vi "Solution part 1.vi"(11 "data?":bool) -> (3 "Occupied seats (result)":i16)   [LabVIEW 2020]
panel:
  out "Rounds":i32
  out "Seats":string[](array[string])
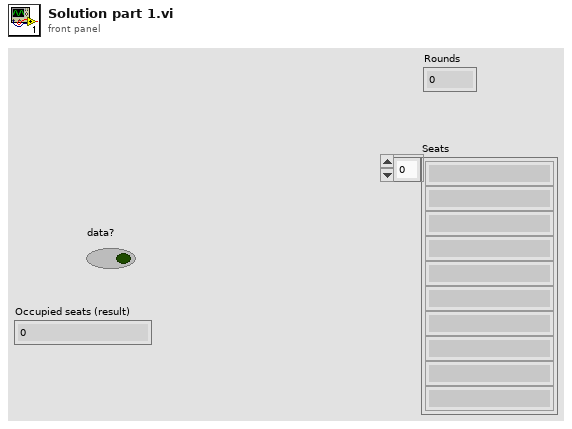
[diagram p1: front panel]
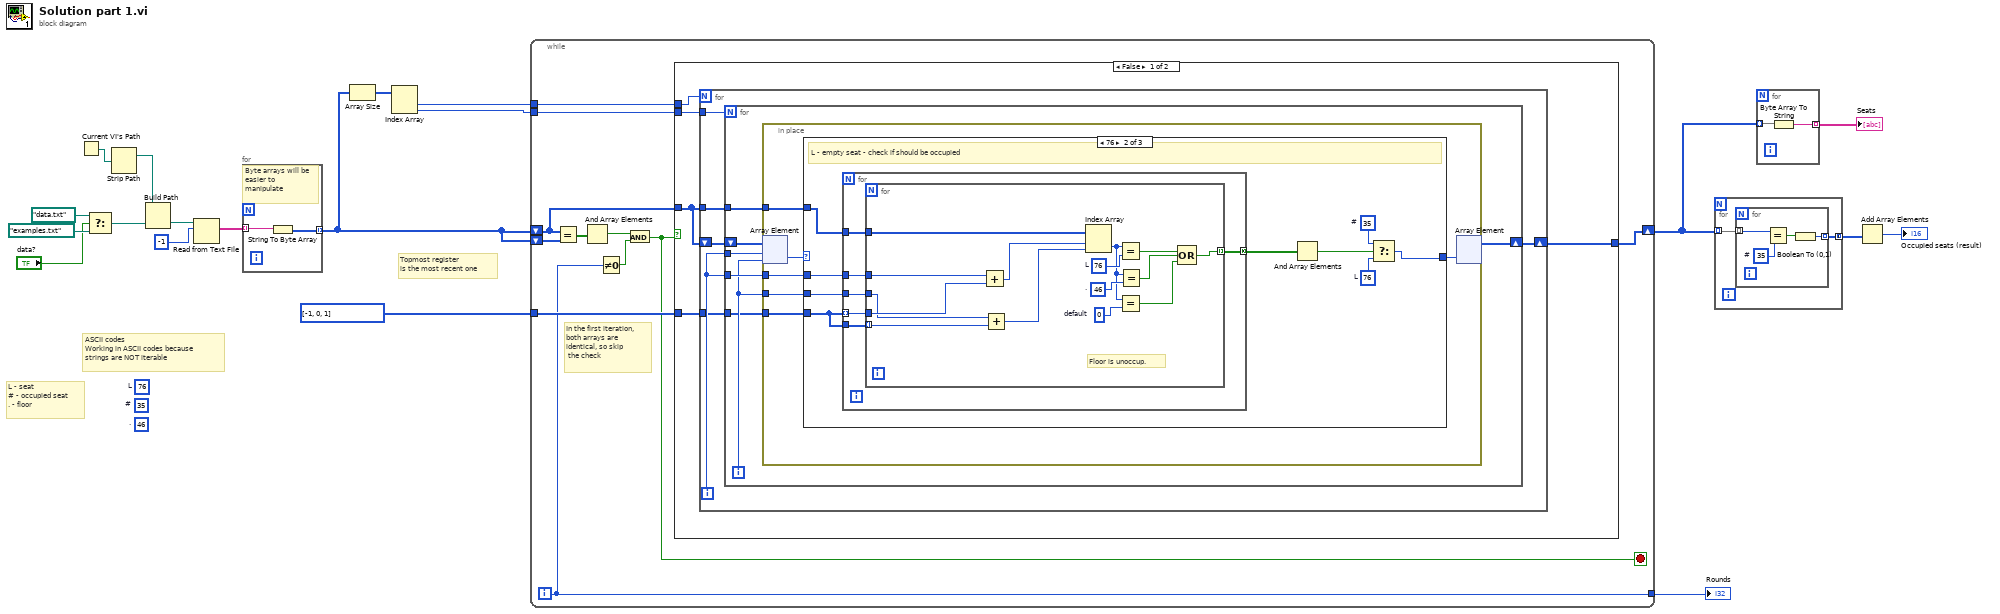
[diagram p0: block diagram]
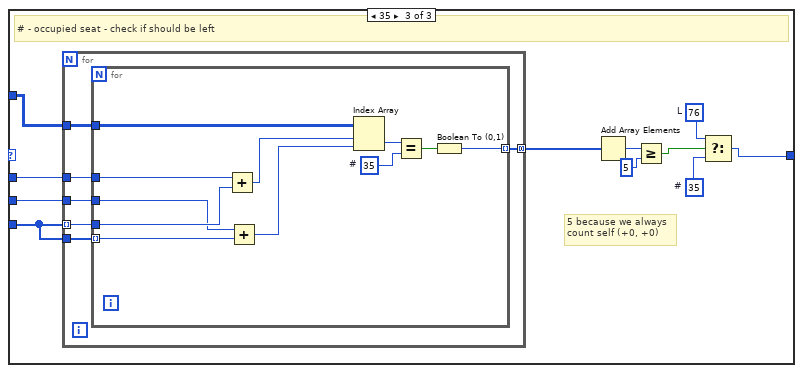
[diagram p3: hidden frame]
diagram:
  (unwired) u8 76  # L
  (unwired) u8 46  # .
  (unwired) u8 35  # #
  # "ASCII codes\nWorking in ASCII codes because\nstrings are NOT iterable"
  # "Topmost register\nis the most recent one"
  # "L - seat\n# - occupied seat\n. - floor"
  n1 = Current VI's Path() -> (path=w16:path)
  n2 = Select(t=path "data.txt", s="data?", f=path "examples.txt") -> (s? t:f=w17:path)
  n3 = Strip Path(path=w16) -> (stripped path=w15:path)  [unwired: 1 out]
  n4 = Build Path(base path=w15, name or relative path=w17) -> (appended path=w14:path)
  n5 = Read from Text File(file (use dialog)=w14, count=-1) -> (text=w11:string[])  [unwired: 2 in, 3 out]
  n6 = for {
    tunnel: w11 -> [w21] mode=indexing
    tunnel: [w20] -> w2 mode=indexing
    # "Byte arrays will be easier to manipulate"
    n7 = String To Byte Array(string=w21) -> (unsigned byte array=w20:u8[])
  }
  n8 = Array Size(array=w2) -> (size(s)=w10:i32[])
  n9 = Index Array(array=w10) -> (element #1=w5:i32, element #2=w6:i32)  [unwired: 2 in]
  n10 = while {
    shift-right: [w30] -> w4
    shift-left: w2 -> [w31]
    shift-left: w2 -> [w22]
    tunnel: w5 -> [w29]
    tunnel: w6 -> [w28]
    tunnel: i32[] [-1, 0, 1] -> [w27]
    tunnel: [w23] -> w1
    i -> [w23]
    stop <- w25 stop-if-true
    # "In the first iteration,\nboth arrays are \nidentical, so skip\n the check"
    n11 = Equal?(x=w22, y=w31) -> (x = y?=w32:bool[][])
    n12 = And Array Elements(Boolean array=w32) -> (logical AND=w26:bool)
    n13 = Not Equal To 0?(x=w23) -> (x != 0?=w24:bool)
    n14 = And(x=w26, y=w24) -> (x .and. y?=w25:bool)
    n15 = case shown="False" w25 {
      tunnel: w22 -> [w33 w116]
      tunnel: [w37 w116] -> w30
      tunnel: w29 -> [w35 _]
      tunnel: w28 -> [w34 _]
      tunnel: w27 -> [w36 _]
      frame False {
        n16 = for {
          N: w35 -> [_]
          tunnel: w34 -> [w42]
          shift-right: [w41] -> w37
          shift-left: w33 -> [w43]
          tunnel: w36 -> [w39]
          tunnel: w33 -> [w38]
          i -> [w40]
          n17 = for {
            N: w42 -> [_]
            tunnel: w40 -> [w50]
            shift-right: [w49] -> w41
            shift-left: w43 -> [w48]
            tunnel: w40 -> [w47]
            tunnel: w39 -> [w45]
            tunnel: w38 -> [w44]
            i -> [w46]
            n18 = in-place {
              in-place-border: w44 -> [w54]
              in-place-border: w47 -> [w53]
              in-place-border: w46 -> [w52]
              in-place-border: w45 -> [w51]
              n19 = in-place-array #1(w48, w50, w46) -> (w56:u8)
              n20 = case shown="76" w56 {
                selector: w56 -> [w57 _ _]
                tunnel: [w57 w58 w94] -> w55
                tunnel: w54 -> [_ w65 w97]
                tunnel: w53 -> [_ w64 w96]
                tunnel: w52 -> [_ w63 w95]
                tunnel: w51 -> [_ w66 w98]
                frame 46, Default {
                  # ". - Floor - skip"
                }
                frame 76 {
                  w59 = u8 35  # #
                  w60 = u8 76  # L
                  # "L - empty seat - check if should be occupied"
                  n21 = for {
                    tunnel: w66 -> [w72] mode=indexing
                    tunnel: w66 -> [w71]
                    tunnel: w65 -> [w70]
                    tunnel: w64 -> [w69]
                    tunnel: w63 -> [w68]
                    tunnel: [w67] -> w62 mode=concatenating
                    n22 = for {
                      tunnel: w72 -> [w83]
                      tunnel: w71 -> [w85] mode=indexing
                      tunnel: w70 -> [w87]
                      tunnel: w69 -> [w86]
                      tunnel: w68 -> [w82]
                      tunnel: [w84] -> w67 mode=indexing
                      w76 = u8 0  # default
                      w75 = u8 46  # .
                      w79 = u8 76  # L
                      # "Floor is unoccup."
                      n23 = Add(x=w86, y=w83) -> (x+y=w81:i32)
                      n24 = Add(x=w82, y=w85) -> (x+y=w80:i32)
                      n25 = Index Array(array=w87, index (row)=w81, index (col)=w80) -> (element=w74:u8)
                      n26 = Equal?(x=w74, y=w79) -> (x = y?=w78:bool)
                      n27 = Equal?(x=w74, y=w76) -> (x = y?=w73:bool)
                      n28 = Equal?(x=w74, y=w75) -> (x = y?=w77:bool)
                      n29 = Compound Arithmetic op=OR(w78, w77, w73) -> (w84:bool)
                    }
                  }
                  n30 = And Array Elements(Boolean array=w62) -> (logical AND=w61:bool)
                  n31 = Select(t=w59, s=w61, f=w60) -> (s? t:f=w58:u8)
                }
                frame 35 {
                  w93 = u8 35  # #
                  w92 = u8 76  # L
                  # "5 because we always\ncount self (+0, +0)"
                  # "# - occupied seat - check if should be left"
                  n32 = for {
                    tunnel: w98 -> [w104] mode=indexing
                    tunnel: w98 -> [w103]
                    tunnel: w97 -> [w102]
                    tunnel: w96 -> [w101]
                    tunnel: w95 -> [w100]
                    tunnel: [w99] -> w91 mode=concatenating
                    n33 = for {
                      tunnel: w104 -> [w114]
                      tunnel: w103 -> [w111] mode=indexing
                      tunnel: w102 -> [w115]
                      tunnel: w101 -> [w113]
                      tunnel: w100 -> [w112]
                      tunnel: [w105] -> w99 mode=indexing
                      w107 = u8 35  # #
                      n34 = Add(x=w113, y=w114) -> (x+y=w110:i32)
                      n35 = Add(x=w112, y=w111) -> (x+y=w109:i32)
                      n36 = Index Array(array=w115, index (row)=w110, index (col)=w109) -> (element=w108:u8)
                      n37 = Equal?(x=w108, y=w107) -> (x = y?=w106:bool)
                      n38 = Boolean To (0,1)(Boolean=w106) -> (0, 1=w105:i16)
                    }
                  }
                  n39 = Add Array Elements(numeric array=w91) -> (sum=w90:i16)
                  n40 = Greater Or Equal?(x=w90, y=i16 5) -> (x >= y?=w88:bool)
                  n41 = Select(t=w92, s=w88, f=w93) -> (s? t:f=w94:u8)
                }
              }
              n42 = in-place-array #1(w55) -> (w49:u8[][])  [unwired: 2 out]
            }
          }
        }
      }
      frame True {
      }
    }
  }
  "Rounds" <- w1
  n43 = for {
    tunnel: w4 -> [w118] mode=indexing
    tunnel: [w117] -> w8 mode=concatenating
    n44 = for {
      tunnel: w118 -> [w122] mode=indexing
      tunnel: [w120] -> w117 mode=indexing
      w119 = u8 35  # #
      n45 = Equal?(x=w122, y=w119) -> (x = y?=w121:bool)
      n46 = Boolean To (0,1)(Boolean=w121) -> (0, 1=w120:i16)
    }
  }
  n47 = for {
    tunnel: w4 -> [w124] mode=indexing
    tunnel: [w123] -> w3 mode=indexing
    n48 = Byte Array To String(unsigned byte array=w124) -> (string=w123:string)
  }
  "Seats" <- w3
  n49 = Add Array Elements(numeric array=w8) -> (sum=→"Occupied seats (result)":i16)
